vi "Write Active Funnel.vi"(8 "error in (no error)":errorcluster, 10 "Active Funnel":refnum<class "Funnel Settings.lvclass">, 11 "Setting Database in":refnum<class "Setting Database.lvclass">) -> (0 "error out":errorcluster, 3 "Setting Database out":refnum<class "Setting Database.lvclass">)   [LabVIEW 2019, in "Setting Database.lvclass"]
uses:
  Setting Database.lvclass
  Funnel Settings/Funnel Settings.lvclass
  C:/Users/Albro/Documents/GitHub/AFM-Lithography/lvsrc/Classes/Settings/ObjectSettings/ObjectSettings.lvclass
  Setting Database.lvclass/Setting Database.ctl
  ObjectSettings/ObjectSettings.lvclass/ObjectSettings.ctl
  ObjectSettings/Accessors/Read Enabled.vi
  ObjectSettings/Accessors/Write Enabled.vi
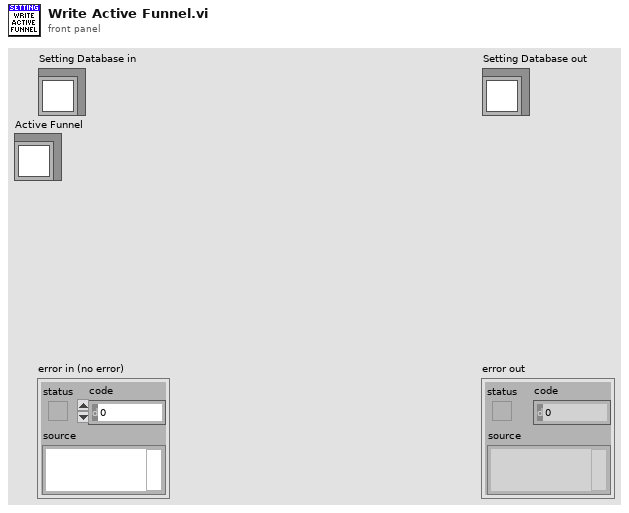
[diagram p1: front panel]
types:
  T1 = cluster{"Path":i32, "Funnel":i32, "Rectangle":i32, "Dot":i32}
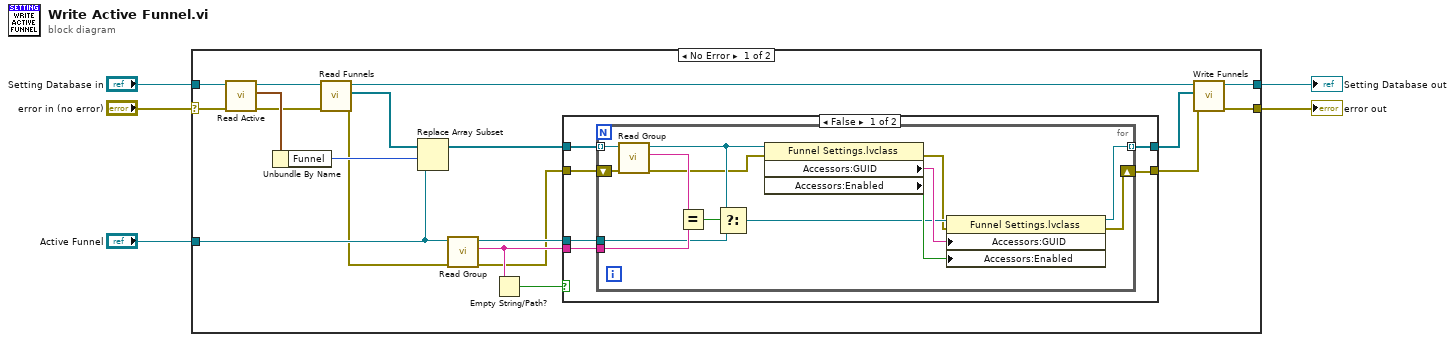
[diagram p0: block diagram]
diagram:
  n1 = case shown="No Error" "error in (no error)" {
    selector: "error in (no error)" -> [w24 w48]
    tunnel: [w6 w48] -> w1
    tunnel: [w9 w47] -> w2
    tunnel: "Setting Database in" -> [w23 w47]
    tunnel: "Active Funnel" -> [w20 _]
    frame No Error {
      n2 = call "Read Active.vi"("error in (no error)"=w24, "Setting Database in"=w23) -> ("error out"=w11:errorcluster, "Active"=w22:T1, "Setting Database out"=w14:refnum<class "Setting Database.lvclass">)  [unwired: 7 in]
      n3 = Unbundle By Name(w22) -> ("Funnel"=w21:i32)
      n4 = call "Read Funnels.vi"("error in (no error)"=w11, "Setting Database in"=w14) -> ("error out"=w12:errorcluster, "Funnels"=w13:refnum<class "Funnel Settings.lvclass">[], "Setting Database out"=w10:refnum<class "Setting Database.lvclass">)  [unwired: 7 in]
      n5 = Replace Array Subset(array=w13, new element=w20, index=w21) -> (w19:refnum<class "Funnel Settings.lvclass">[])
      n6 = call-dynamic "Read Group.vi"("error in (no error)"=w12, "ObjectSettings in"=w20) -> ("error out"=w15:errorcluster, "Group"=w17:string, "ObjectSettings out"=w16:refnum<class "Funnel Settings.lvclass">)  [unwired: 7 in]
      n7 = Empty String/Path?(string/path=w17) -> (empty?=w18:bool)
      n8 = case shown="False" w18 {
        tunnel: w19 -> [w29 w46]
        tunnel: [w27 w46] -> w8
        tunnel: w17 -> [w30 _]
        tunnel: w16 -> [w28 _]
        tunnel: w15 -> [w26 w45]
        tunnel: [w25 w45] -> w7
        frame False {
          n9 = for {
            tunnel: w30 -> [w42]
            tunnel: w29 -> [w44] mode=indexing
            tunnel: w28 -> [w41]
            tunnel: [w39] -> w27 mode=indexing
            shift-right: [w31] -> w25
            shift-left: w26 -> [w32]
            n10 = call-dynamic "Read Group.vi"("error in (no error)"=w32, "ObjectSettings in"=w44) -> ("error out"=w33:errorcluster, "Group"=w43:string, "ObjectSettings out"=w40:refnum<class "Funnel Settings.lvclass">)  [unwired: 7 in]
            n11 = Equal?(x=w43, y=w42) -> (x = y?=w35:bool)
            n12 = Select(t=w40, s=w35, f=w41) -> (s? t:f=w36:refnum<class "Funnel Settings.lvclass">)
            n13 = property class="Funnel Settings.lvclass"(reference=w40, error in=w33) -> (error out=w34:errorcluster, "Accessors:GUID"=w38:string, "Accessors:Enabled"=w37:bool)  [unwired: 1 out]
            n14 = property class="Funnel Settings.lvclass"(reference=w36, error in=w34, "Accessors:GUID"=w38, "Accessors:Enabled"=w37) -> (reference out=w39:refnum<class "Funnel Settings.lvclass">, error out=w31:errorcluster)
          }
        }
        frame True {
        }
      }
      n15 = call "Write Funnels.vi"("error in (no error)"=w7, "Funnels"=w8, "Setting Database in"=w10) -> ("error out"=w6:errorcluster, "Setting Database out"=w9:refnum<class "Setting Database.lvclass">)  [unwired: 7 in]
    }
    frame Error {
    }
  }
  "error out" <- w1
  "Setting Database out" <- w2
